vi "Adjust_Test_Signal_Level_popup.vi"() -> ()   [LabVIEW 2020]
panel:
  out "Select Multiplier and Click OK 2":T1(radio)
  in  "Cancel Button":bool
  in  "OK Button":bool
  in  "Select Multiplier and Click OK":T1(radio)
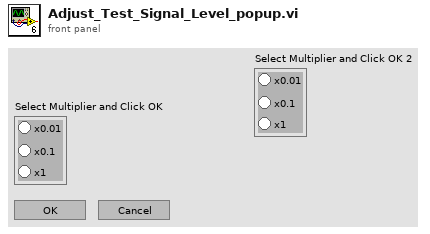
[diagram p1: front panel]
types:
  T1 = enum32{"No Selection", "TestSigLevx0.01", "TestSigLevx0.1", "TestSigLevx1"}
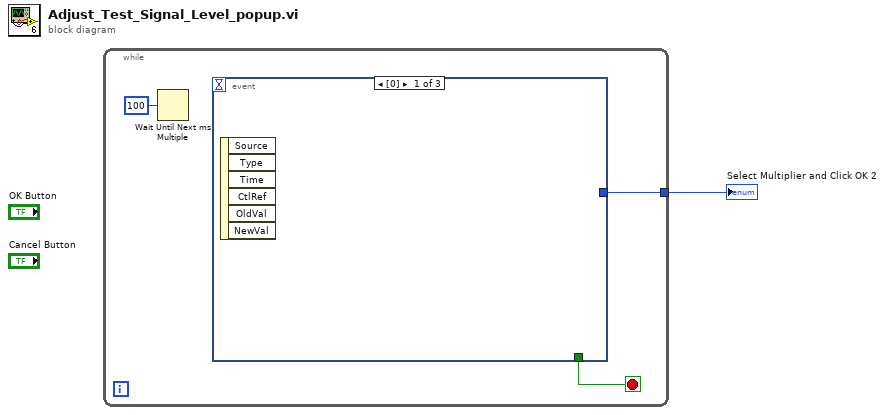
[diagram p0: block diagram]
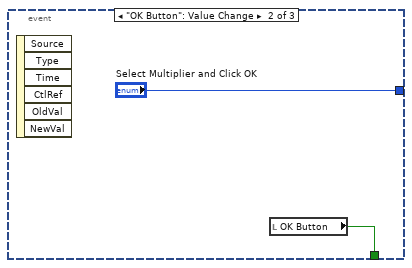
[diagram p2: hidden frame]
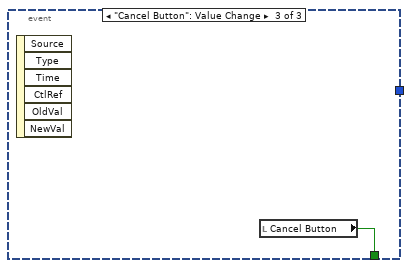
[diagram p3: hidden frame]
diagram:
  n1 = while {
    tunnel: [w3] -> w1
    stop <- w2 stop-if-true
    n2 = Wait Until Next ms Multiple(millisecond multiple=u32 100) -> ()  [unwired: 1 out]
    n3 = event shown="[0]" {
      selector: _ -> [_ _ _]
      dyn-events: _ -> [_ _ _]
      timeout: _ -> [_ _ _]
      tunnel: [_ "Select Multiplier and Click OK" _] -> w3
      tunnel: [_ w5 w7] -> w2
      event #0 (no event record) {
        n4 = event-data() -> ()  [unwired: 1 in, 6 out]
      }
      event "OK Button": Value Change {
        n5 = event-data() -> ()  [unwired: 1 in, 6 out]
        n6 = local read "OK Button"() -> (w5:bool)
      }
      event "Cancel Button": Value Change {
        n7 = event-data() -> ()  [unwired: 1 in, 6 out]
        n8 = local read "Cancel Button"() -> (w7:bool)
      }
    }
  }
  "Select Multiplier and Click OK 2" <- w1
